vi "get_mux_pin.vi"(10 "Cell Details Cluster":T1={"Cell Position"=16, "Cell Label"="", "Pixel to measure"=0, "Area (cm^2)"=0.126, "Variable"="", "Variable value"="", "Scan settings in queue"=0, "Light or dark"="", "Measurement Type"=""} {"Pixel to measure" items=["All", "1", "2", "3", "4", "5", "6", "7", "8"]}) -> (0 "Pin":dbl)   [LabVIEW 2016]
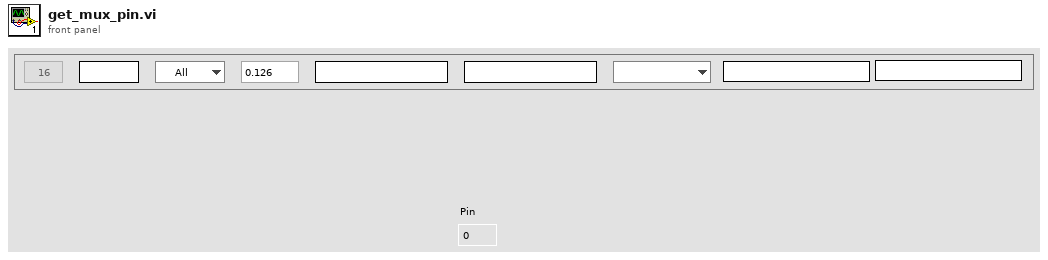
[diagram p1: front panel]
types:
  T1 = cluster{"Cell Position":i32, "Cell Label":string, "Pixel to measure":u16, "Area (cm^2)":dbl, "Variable":string, "Variable value":string, "Scan settings in queue":u16, "Light or dark":string, "Measurement Type":string}
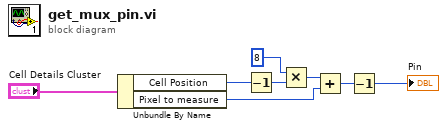
[diagram p0: block diagram]
diagram:
  n1 = Unbundle By Name("Cell Details Cluster") -> ("Cell Position"=w5:i32, "Pixel to measure"=w3:u16)
  n2 = Decrement(x=w5) -> (x-1=w6:i32)
  n3 = Multiply(x=8, y=w6) -> (x*y=w4:i32)
  n4 = Add(x=w4, y=w3) -> (x+y=w2:i32)
  n5 = Decrement(x=w2) -> (x-1=→"Pin":i32)
